vi "FindProgress.vi"(9 "total time (sec)":sgl, 10 "Total Pixels":u64, 11 "Wave Count":u64) -> (2 "TimeString":string, 3 "Progress%":u8)   [LabVIEW 2020]
panel:
  out "Seconds":u8
  out "Mins":u8
  out "Hours":u8
  out "Seconds Remaining":dbl
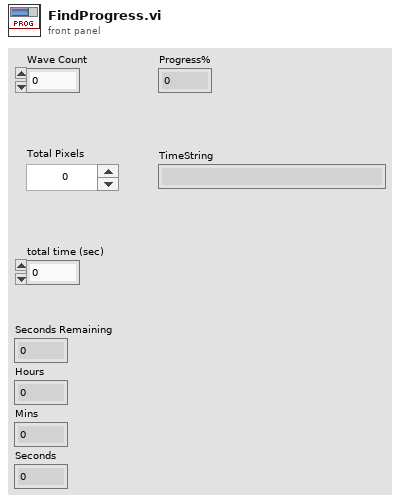
[diagram p1: front panel]
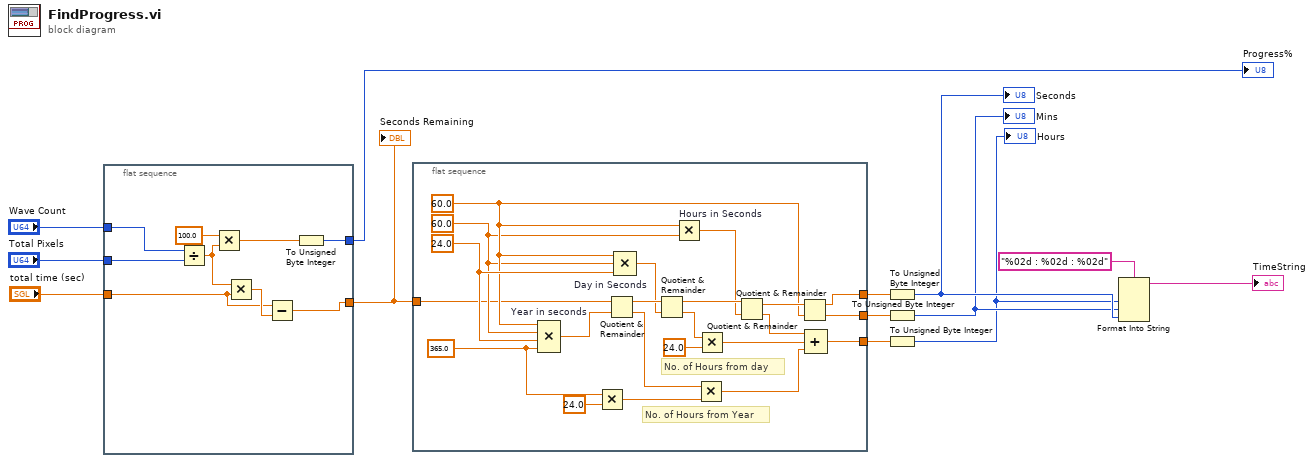
[diagram p0: block diagram]
diagram:
  n1 = flat-sequence {
    tunnel: "Wave Count" -> [w21]
    tunnel: "Total Pixels" -> [w20]
    tunnel: [w19] -> w11
    tunnel: "total time (sec)" -> [w16]
    tunnel: [w15] -> w1
    frame #0 {
      n2 = Divide(x=w21, y=w20) -> (x/y=w14:dbl)
      n3 = Multiply(x=100.0, y=w14) -> (x*y=w18:dbl)
      n4 = Multiply(x=w14, y=w16) -> (x*y=w17:dbl)
      n5 = Subtract(x=w16, y=w17) -> (x-y=w15:dbl)
      n6 = To Unsigned Byte Integer(number=w18) -> (unsigned 8bit integer=w19:u8)
    }
  }
  n7 = flat-sequence {
    tunnel: [w32] -> w8
    tunnel: [w31] -> w7
    tunnel: [w30] -> w6
    tunnel: w1 -> [w23]
    frame #0 {
      w26 = 365.0
      w38 = 24.0
      w28 = 60.0
      w29 = 60.0
      # "No. of Hours from day"
      # "No. of Hours from Year"
      n8 = Compound Arithmetic op=MULTIPLY "Year in seconds"(w29, w28, w38, w26) -> (w44:dbl)
      n9 = Multiply(x=w26, y=24.0) -> (x*y=w24:dbl)
      n10 = Quotient & Remainder(x=w23, y=w44) -> (x-y*floor(x/y)=w43:dbl, floor(x/y)=w40:dbl)
      n11 = Compound Arithmetic op=MULTIPLY "Day in Seconds"(w29, w28, w38) -> (w39:dbl)
      n12 = Quotient & Remainder(x=w43, y=w39) -> (x-y*floor(x/y)=w42:dbl, floor(x/y)=w37:dbl)
      n13 = Multiply "Hours in Seconds"(x=w29, y=w28) -> (x*y=w41:dbl)
      n14 = Multiply(x=w40, y=w24) -> (x*y=w33:dbl)
      n15 = Multiply(x=w37, y=24.0) -> (x*y=w34:dbl)
      n16 = Quotient & Remainder(x=w42, y=w41) -> (x-y*floor(x/y)=w36:dbl, floor(x/y)=w35:dbl)
      n17 = Quotient & Remainder(x=w36, y=w29) -> (x-y*floor(x/y)=w30:dbl, floor(x/y)=w31:dbl)
      n18 = Compound Arithmetic op=ADD(w35, w34, w33) -> (w32:dbl)
    }
  }
  n19 = To Unsigned Byte Integer(number=w6) -> (unsigned 8bit integer=w4:u8)
  "Seconds" <- w4
  n20 = To Unsigned Byte Integer(number=w7) -> (unsigned 8bit integer=w3:u8)
  "Mins" <- w3
  n21 = To Unsigned Byte Integer(number=w8) -> (unsigned 8bit integer=w2:u8)
  "Hours" <- w2
  n22 = Format Into String(format string="%02d : %02d : %02d", w2, w3, w4) -> (resulting string=→"TimeString":string)  [unwired: 2 in, 1 out]
  "Progress%" <- w11
  "Seconds Remaining" <- w1
